vi "TDT-Start.vi"(4 "error in (no error)":errorcluster, 5 "RPcoX":refnum<k7>) -> (0 "error out":errorcluster, 1 "RPcoX out":refnum<k7>)   [LabVIEW 2020]
doc: "Sends <B>Start</B> notifier to DAQ thread to begin measurement."
uses:
  TDT-Signal Bank Action.ctl
  TDT-Globals.vi
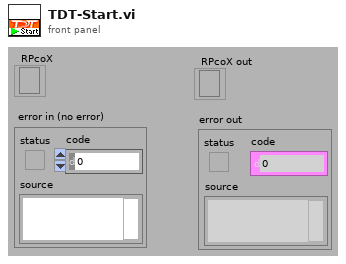
[diagram p1: front panel]
types:
  T1 = typedef "TDT-Signal Bank Action.ctl" = enum16{"Init", "Write", "Read", "Rewrite", "Reset", "Recycle", "Ramp up", "Ramp down", "Zero"}
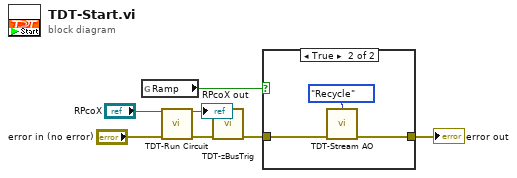
[diagram p0: block diagram]
diagram:
  n1 = global read "TDT-Globals.vi" "Ramp"() -> (w4:bool)
  n2 = call "TDT-Run Circuit.vi"("RPcoX"="RPcoX", "error in (no error)"="error in (no error)") -> ("RPcoX out"=→"RPcoX out":refnum<k7>, "error out"=w7:errorcluster)  [unwired: 12 in]
  n3 = call "TDT-zBusTrig.vi"("error in (no error)"=w7) -> ("error out"=w5:errorcluster)  [unwired: 6 in]
  n4 = case shown="True" w4 {
    tunnel: w5 -> [w8 w11]
    tunnel: [w8 w10] -> w3
    frame False {
    }
    frame True {
      n5 = call "TDT-Stream AO.vi"("Action"=TDT-Signal_Bank_Action."Recycle", "error in (no error)"=w11) -> ("error out"=w10:errorcluster)  [unwired: 12 in, 1 out]
    }
  }
  "error out" <- w3
